vi "Get Database Manager.vi"(8 "error in (no error)":errorcluster, 11 "Objects in":refnum<class "Objects.lvclass">) -> (0 "error out":errorcluster, 2 "Database Manager":refnum<class "Database Manager.lvclass">, 3 "Objects out":refnum<class "Objects.lvclass">)   [LabVIEW 2019, in "HierDAL Library.lvlib" / "Database.lvlib" / "Repositories.lvlib" / "Objects.lvclass"]
uses:
  Objects.lvclass
  Database Manager Class/Database Manager.lvclass
  Objects.lvclass/Objects.ctl
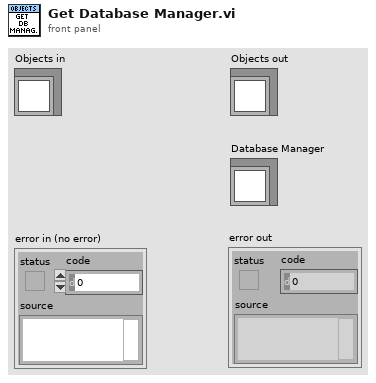
[diagram p1: front panel]
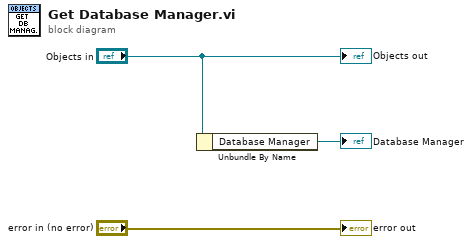
[diagram p0: block diagram]
diagram:
  n1 = Unbundle By Name("Objects in") -> ("Database Manager"=→"Database Manager":refnum<class "Database Manager.lvclass">)
  "error out" <- "error in (no error)"
  "Objects out" <- "Objects in"
